vi "ID .vi"() -> (3 "机器ID":string)   [LabVIEW 2013]
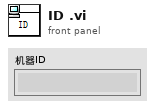
[diagram p1: front panel]
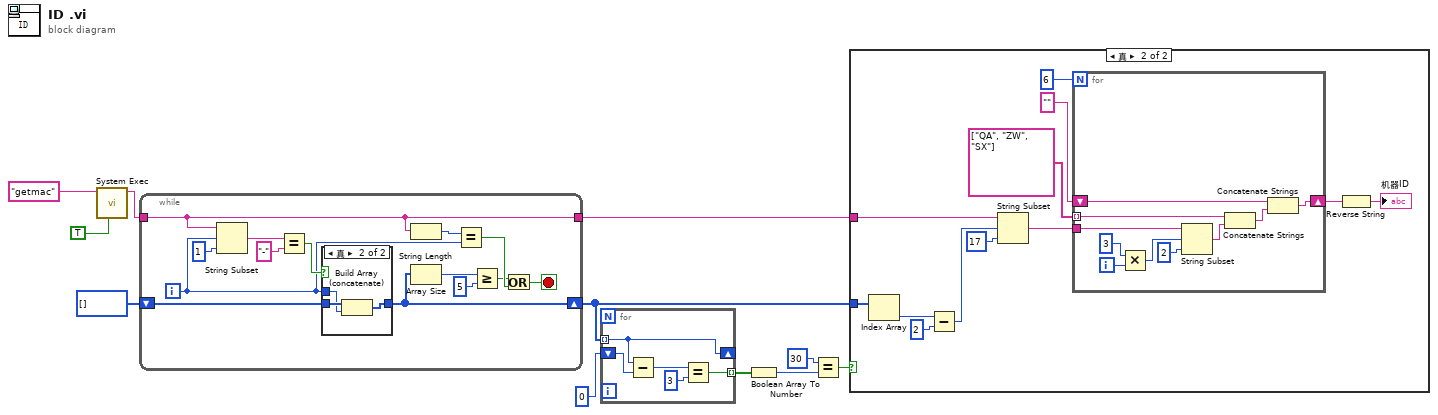
[diagram p0: block diagram]
diagram:
  n1 = call <vilib>:"System Exec.vi"("run minimized? (F)"=TRUE, "command line"="getmac") -> ("standard output"=w9:string)  [unwired: 4 in, 5 out]
  n2 = while {
    tunnel: w9 -> [w12]
    shift-right: [w16] -> w1
    shift-left: i32[] [] -> [w20]
    tunnel: [w12] -> w2
    i -> [w19]
    stop <- w17 stop-if-true
    n3 = String Subset(string=w12, offset (0)=w19, length (rest)=1 ("长度（剩余）")) -> (substring=w24:string)
    n4 = Equal?(x=w24, y="-" ("子字符串(\"\")")) -> (x = y?=w21:bool)
    n5 = case shown="真" w21 {
      tunnel: [w26 w29] -> w16
      tunnel: w20 -> [w26 w28]
      tunnel: w19 -> [_ w27]
      frame False {
      }
      frame True {
        n6 = Build Array (concatenate)(w28, w27) -> (w29:i32[])
      }
    }
    n7 = String Length(string=w12) -> (length=w22:i32)
    n8 = Array Size(array=w16) -> (size(s)=w15:i32)
    n9 = Equal?(x=w22, y=w19) -> (x = y?=w18:bool)
    n10 = Greater Or Equal?(x=w15, y=5) -> (x >= y?=w13:bool)
    n11 = Or(x=w13, y=w18) -> (x .or. y?=w17:bool)
  }
  n12 = for {
    tunnel: w1 -> [w31] mode=indexing
    shift-right: [w31] -> _
    shift-left: 0 -> [w30]
    tunnel: [w32] -> w6 mode=indexing
    n13 = Subtract(x=w31, y=w30) -> (x-y=w34:i32)
    n14 = Equal?(x=w34, y=3) -> (x = y?=w32:bool)
  }
  n15 = Boolean Array To Number(Boolean array=w6) -> (number=w5:u32)
  n16 = Equal?(x=u32 30, y=w5) -> (x = y?=w3:bool)
  n17 = case shown="真" w3 {
    tunnel: w2 -> [_ w43]
    tunnel: w1 -> [_ w46]
    frame False {
    }
    frame True {
      n18 = Index Array(array=w46) -> (element=w45:i32)  [unwired: 1 in]
      n19 = Subtract(x=w45, y=2) -> (x-y=w42:i32)
      n20 = String Subset(string=w43, offset (0)=w42, length (rest)=17 ("长度（剩余）")) -> (substring=w39:string)
      n21 = for {
        N: 6 -> [_]
        tunnel: w39 -> [w56]
        tunnel: string[] ["QA", "ZW", "SX"] -> [w51] mode=indexing
        shift-right: [w48] -> w36
        shift-left: "" -> [w50]
        i -> [w55]
        n22 = Multiply(x=3, y=w55) -> (x*y=w53:i32)
        n23 = String Subset(string=w56, offset (0)=w53, length (rest)=2 ("长度（剩余）")) -> (substring=w52:string)
        n24 = Concatenate Strings(w51, w52) -> (w49:string)
        n25 = Concatenate Strings(w50, w49) -> (w48:string)
      }
      n26 = Reverse String(1:w36) -> (0:→"机器ID":string)
    }
  }
